vi "PID360.vi"(10 "Yaw":dbl, 11 "Angle":dbl) -> (3 "Numeric":dbl)   [LabVIEW 2015]
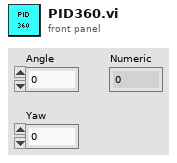
[diagram p1: front panel]
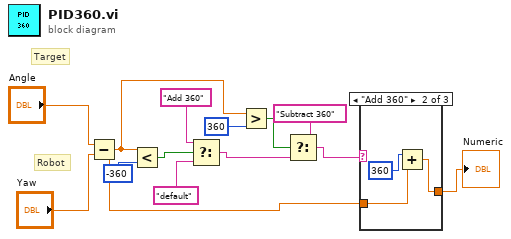
[diagram p0: block diagram]
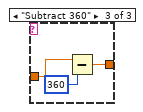
[diagram p3: hidden frame]
diagram:
  # "Robot"
  # "Target"
  n1 = Subtract(x="Angle", y="Yaw") -> (x-y=w2:dbl)
  n2 = Less?(x=w2, y=-360) -> (x < y?=w5:bool)
  n3 = Select(t="Add 360", s=w5, f="default") -> (s? t:f=w7:string)
  n4 = Greater?(x=w2, y=360) -> (0:w6:bool)
  n5 = Select(t="Subtract 360", s=w6, f=w7) -> (s? t:f=w3:string)
  n6 = case shown="\"Add 360\"" w3 {
    tunnel: w2 -> [w14 w16 w19]
    tunnel: [w14 w15 w18] -> w1
    frame "default", Default {
    }
    frame "Add 360" {
      n7 = Add(x=360, y=w16) -> (x+y=w15:dbl)
    }
    frame "Subtract 360" {
      n8 = Subtract(x=w19, y=360) -> (x-y=w18:dbl)
    }
  }
  "Numeric" <- w1
